vi "836_CameraSend Images To PC Loop.vi"(6 "Video Mode":i32, 8 "error in (no error)":errorcluster, 9 "fps":u16, 10 "port":u16=1180, 11 "CameraDevRef":T1) -> (0 "error IO":errorcluster)   [LabVIEW 2015]
doc: "This VI is used to send images to the dashboard using the second enet port on the 8 slot controller. This is provided for compatibility, but is higher overhead than using the Camera MJPG approach.\n\nThis software is licensed. Open the labview\\readme\\WPI Robotics Library Open Source License.txt file for more information."
uses:
  <vilib>/Rock Robotics/WPI/Camera/WPI_CameraDevRef.ctl
  <vilib>/Rock Robotics/SystemInterfaces/NetworkCommunication/NetComm_UsageReport_ResourceType.ctl
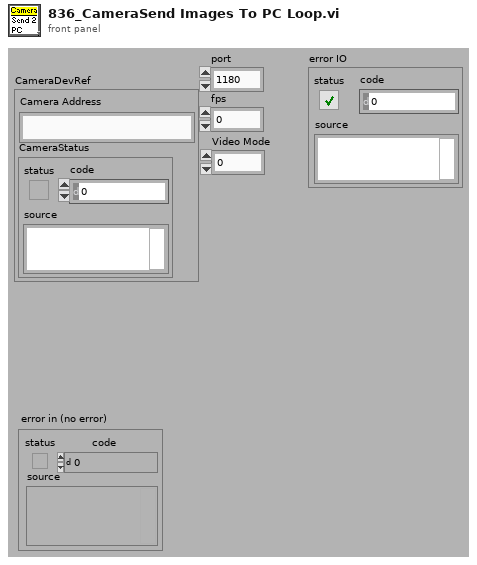
[diagram p1: front panel]
types:
  T1 = typedef "WPI_CameraDevRef.ctl" = cluster{"Camera Address":string, "CameraStatus":errorcluster}
  T2 = typedef "NetComm_UsageReport_ResourceType.ctl" = enum8{"Controller", "Module", "Language", "CANPlugin", "Accelerometer", "ADXL345", "AnalogChannel", "AnalogTrigger", "AnalogTriggerOutput", "CANJaguar", "Compressor", "Counter", "Dashboard", "DigitalInput", "DigitalOutput", "DriverStationCIO", "DriverStationEIO", "DriverStationLCD", "Encoder", "GearTooth", "Gyro", "I2C", "Framework", "Jaguar", "Joystick", "Kinect", "KinectStick", "PIDController", "Preferences", "PWM", "Relay", "RobotDrive", "SerialPort", "Servo", "Solenoid", "SPI", "Task", "Ultrasonic", "Victor", "Button", "Command", "AxisCamera", "PCVideoServer", "SmartDashboard", "Talon", "HiTechnicColorSensor", "HiTechnicAccel", "HiTechnicCompass", "SRF08", "AnalogOutput", "Victor SP", "Talon SRX", "CAN Talon SRX", "ADXL362 Accel", "ADXRS450 Gyro", "Rev SPARK", "Mindsensors SD540", "Digital Filter"}
  T3 = enum16{"Update Mode", "Get Image", "Get Image Data"}
  T4 = typedef "Image Type" = u32
  T5 = typedef "IMAQ Image.ctl" = refnum<image>
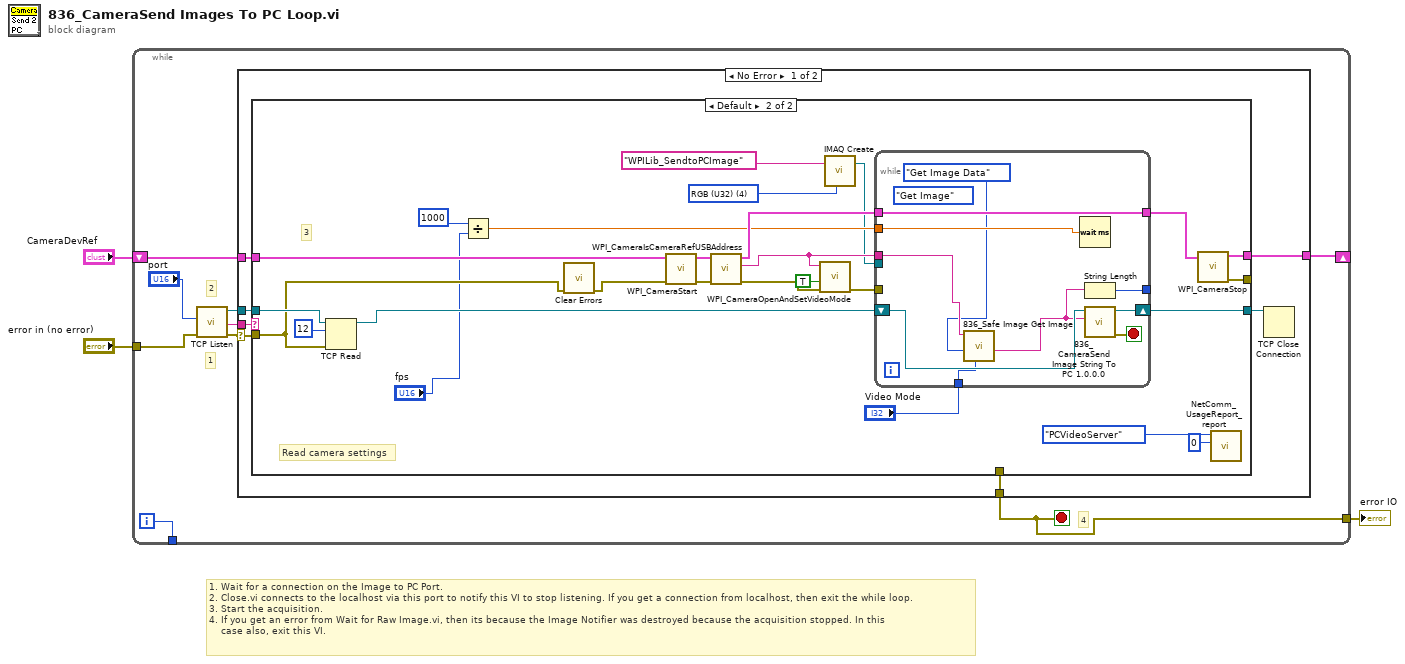
[diagram p0: block diagram]
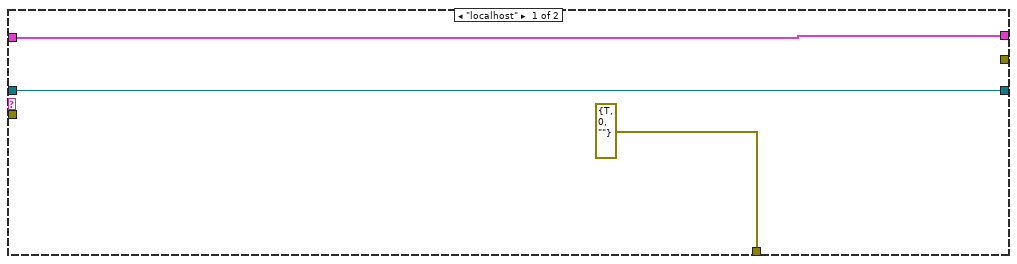
[diagram p2: hidden frame]
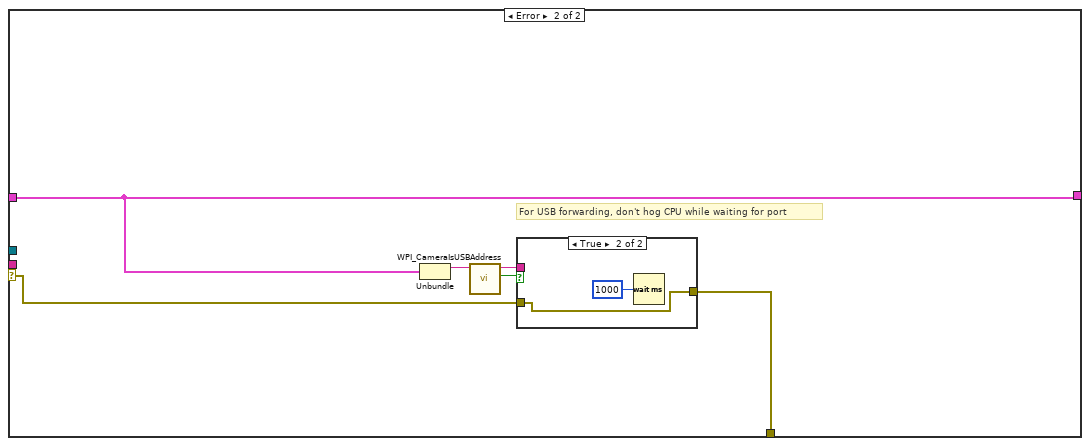
[diagram p3: hidden frame]
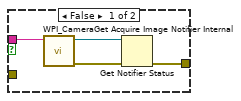
[diagram p4: hidden frame]
diagram:
  # "1. Wait for a connection on the Image to PC Port.\n2. Close.vi connects to the localhost via this port to notify this VI to stop listening. If you get a connection from localhost, then exit the while loop.\n3. Start the acquisition.\n4. If you get an error from Wait for Raw Image.vi, then its because the Image Notifier was destroyed because the acquisition stopped. In this\n    case also, exit this VI."
  n1 = while {
    tunnel: "error in (no error)" -> [w9]
    shift-right: [w12] -> _
    shift-left: "CameraDevRef" -> [w10]
    tunnel: [w5] -> _
    tunnel: [w4] -> w1
    i -> [w5]
    stop <- w4 stop-if-true
    # "4"
    # "1"
    # "2"
    n2 = call <vilib>:"TCP Listen.vi"("error in (no error)"=w9, "port"="port") -> ("error out"=w6:errorcluster, "remote address"=w11:string, "connection ID"=w8:refnum<k5>)  [unwired: 2 in, 5 out]
    n3 = case shown="No Error" w6 {
      selector: w6 -> [w13 w59]
      tunnel: [w19 w63] -> w12
      tunnel: w11 -> [w18 _]
      tunnel: w10 -> [w17 w63]
      tunnel: w8 -> [w16 _]
      tunnel: [w15 w64] -> w4
      frame No Error {
        n4 = case shown="Default" w18 {
          tunnel: [w22 w47] -> w19
          tunnel: w17 -> [w22 w29]
          tunnel: w13 -> [_ w30]
          tunnel: w16 -> [w20 w35]
          tunnel: [errorcluster {"status"=TRUE, "code"=0, "source"=""} ("error out 2") _] -> w15
          tunnel: [w20 w48] -> w14
          tunnel: [_ w46] -> _
          frame "localhost" {
          }
          frame Default {
            w41 = T4 4 items=["Grayscale (U8)", "Grayscale (I16)", "Grayscale (SGL)", "Complex (CSG)", "RGB (U32)", "HSL (U32)", "RGB (U64)", "Grayscale (U16)"] ("Image Type")
            # "Read camera settings"
            # "3"
            n5 = TCP Read(connection ID=w35, bytes to read=12, error in (no error)=w30) -> (connection ID out=w34:refnum<k5>)  [unwired: 2 in, 2 out]
            n6 = Divide(x=u16 1000 ("port"), y="fps") -> (x/y=w31:dbl)
            n7 = call <vilib>:"Clear Errors.vi"("error in (no error)"=w30) -> ("error out"=w28:errorcluster)  [unwired: 5 in, 1 out]
            n8 = call <vilib>:"WPI_CameraStart.vi"("error in (no error)"=w28, "CameraDevRef"=w29) -> ("error out"=w39:errorcluster, "CameraDevRef"=w37:T1)  [unwired: 8 out]
            n9 = call <vilib>:"WPI_CameraIsCameraRefUSBAddress.vi"("error in (no error)"=w39, "CameraDevRef"=w37) -> ("error out"=w38:errorcluster, "Camera Address Out"=w40:string, "CameraDevRef out"=w36:T1)  [unwired: 6 in, 1 out]
            n10 = call <vilib>:"WPI_CameraOpenAndSetVideoMode.vi"("error in (no error)"=w38, "USB JPEG"=TRUE, "Camera Address Out"=w40) -> ("error out"=w26:errorcluster)  [unwired: 8 in]
            n11 = call "IMAQ Create"("Image Name"="WPILib_SendtoPCImage", "Image Type"=w41) -> ("New Image"=w27:T5)  [unwired: 3 in, 1 out]
            n12 = while {
              tunnel: w40 -> [w52]
              shift-right: [w58] -> w48
              shift-left: w34 -> [w54]
              tunnel: w27 -> [_]
              tunnel: [w56] -> w45
              tunnel: w36 -> [w56]
              tunnel: w31 -> [w55]
              tunnel: [w53] -> _
              tunnel: w26 -> [_]
              tunnel: "Video Mode" -> [w49]
              stop <- w57 stop-if-true
              (unwired) T3."Get Image" ("Operation")
              n13 = call "836_Safe Image Get Image.vi"("Video Mode"=w49, "Operation"=T3."Get Image Data", "Session In"=w52) -> ("Image Data String"=w50:string)  [unwired: 5 in, 3 out]
              n14 = Wait (ms)(milliseconds to wait=w55) -> ()  [unwired: 1 out]
              n15 = String Length(string=w50) -> (length=w53:i32)
              n16 = call "836_CameraSend Image String To PC 1.0.0.0.vi"("String"=w50, "TCP Connection ID"=w54) -> ("error out"=w57:errorcluster, "TCP Connection ID out"=w58:refnum<k5>)  [unwired: 8 in]
            }
            n17 = call <vilib>:"WPI_CameraStop.vi"("CameraDevRef"=w45) -> ("error out"=w46:errorcluster, "CameraDevRef"=w47:T1)  [unwired: 1 in, 8 out]
            n18 = call <vilib>:"NetComm_UsageReport_report.vi"("Instance Number"=u8 0, "Resource Type"=NetComm_UsageReport_ResourceType."PCVideoServer") -> ()  [unwired: 10 in]
          }
        }
        n19 = TCP Close Connection(connection ID=w14) -> ()  [unwired: 1 in, 3 out]
      }
      frame Error {
        # "For USB forwarding, don't hog CPU while waiting for port"
        n20 = Unbundle(w63) -> ("Camera Address"=w62:string)  [unwired: 1 out]
        n21 = call <vilib>:"WPI_CameraIsUSBAddress.vi"("Camera Address In"=w62) -> ("USB?"=w60:bool, "Camera Address Out"=w61:string)  [unwired: 8 in, 1 out]
        n22 = case shown="True" w60 {
          tunnel: [w68 w69] -> w64
          tunnel: w61 -> [w65 _]
          tunnel: w59 -> [_ w69]
          frame False {
            n23 = call <vilib>:"WPI_CameraGet Acquire Image Notifier Internal.vi"("Camera Address"=w65) -> ("error out"=w66:errorcluster, "Acquire Image Notifier"=w67:refnum<notifier>)  [unwired: 1 in, 8 out]
            n24 = Get Notifier Status(notifier=w67, error in (no error)=w66) -> (error out=w68:errorcluster)  [unwired: 4 out]
          }
          frame True {
            n25 = Wait (ms)(milliseconds to wait=u32 1000) -> ()  [unwired: 1 out]
          }
        }
      }
    }
  }
  "error IO" <- w1
